vi "Retrieve Question.vi"(8 "error in (no error)":errorcluster, 9 "Difficulty":u32, 10 "Category":string, 11 "Controller in":refnum<class "Controller.lvclass">) -> (0 "error out":errorcluster, 3 "Controller out":refnum<class "Controller.lvclass">)   [LabVIEW 2024, in "Controller.lvlib" / "Controller.lvclass"]
uses:
  Controller.lvclass
  C:/Program Files/National Instruments/LabVIEW 2024/vi.lib/ActorFramework/Actor/Actor.lvclass
  Controller.lvclass/Controller.ctl
  MC Prompt/MC Prompt/MC Prompt.lvclass
  <vilib>/ActorFramework/Actor/Actor.lvclass/Actor.ctl
  <vilib>/ActorFramework/Message Enqueuer/Message Enqueuer.lvclass/Message Enqueuer.ctl
  MC Prompt/MC Prompt/MC Prompt.lvclass/MC Prompt.ctl
  Controller Messages/Question Prompt Display Msg/Question Prompt Display Msg.lvclass/Question Prompt Display Msg.ctl
  MC Screen/Grid Screen Messages/Ensure Cell is Off Msg/Ensure Cell is Off Msg.lvclass/Ensure Cell is Off Msg.ctl
  d7edfcb4-d505-b941-a124-b7699e1ba89e.vi
  <vilib>/ActorFramework/Message Enqueuer/Enqueue.vi
  <vilib>/ActorFramework/Message Enqueuer/Init from Existing Queue.vi
  <vilib>/ActorFramework/Stop Msg/Stop Msg.lvclass
  C:/Program Files/National Instruments/LabVIEW 2024/vi.lib/ActorFramework/Message/Message.lvclass
  Controller Messages/Question Prompt Display Msg/Question Prompt Display Msg.lvclass
  MC Screen/Grid Screen Messages/Ensure Cell is Off Msg/Ensure Cell is Off Msg.lvclass
  <vilib>/ActorFramework/Message Priority Queue/Priority Enqueue.vi
  <vilib>/ActorFramework/Message Enqueuer/Message Enqueuer.lvclass
  <vilib>/ActorFramework/Actor/Actor.lvclass
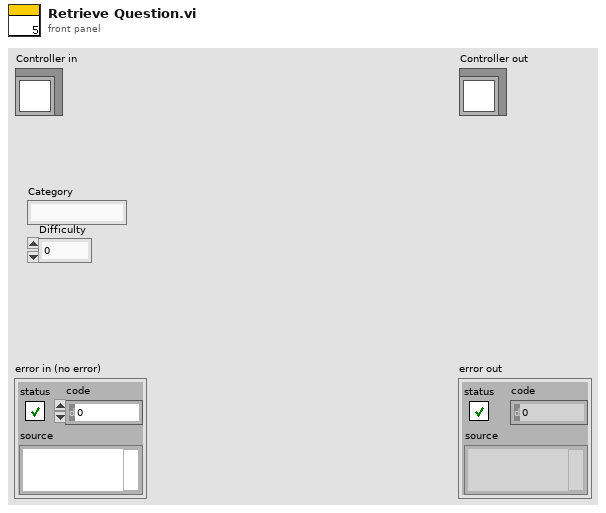
[diagram p1: front panel]
types:
  T1 = map{cluster{"String":string, "String":string}, path}
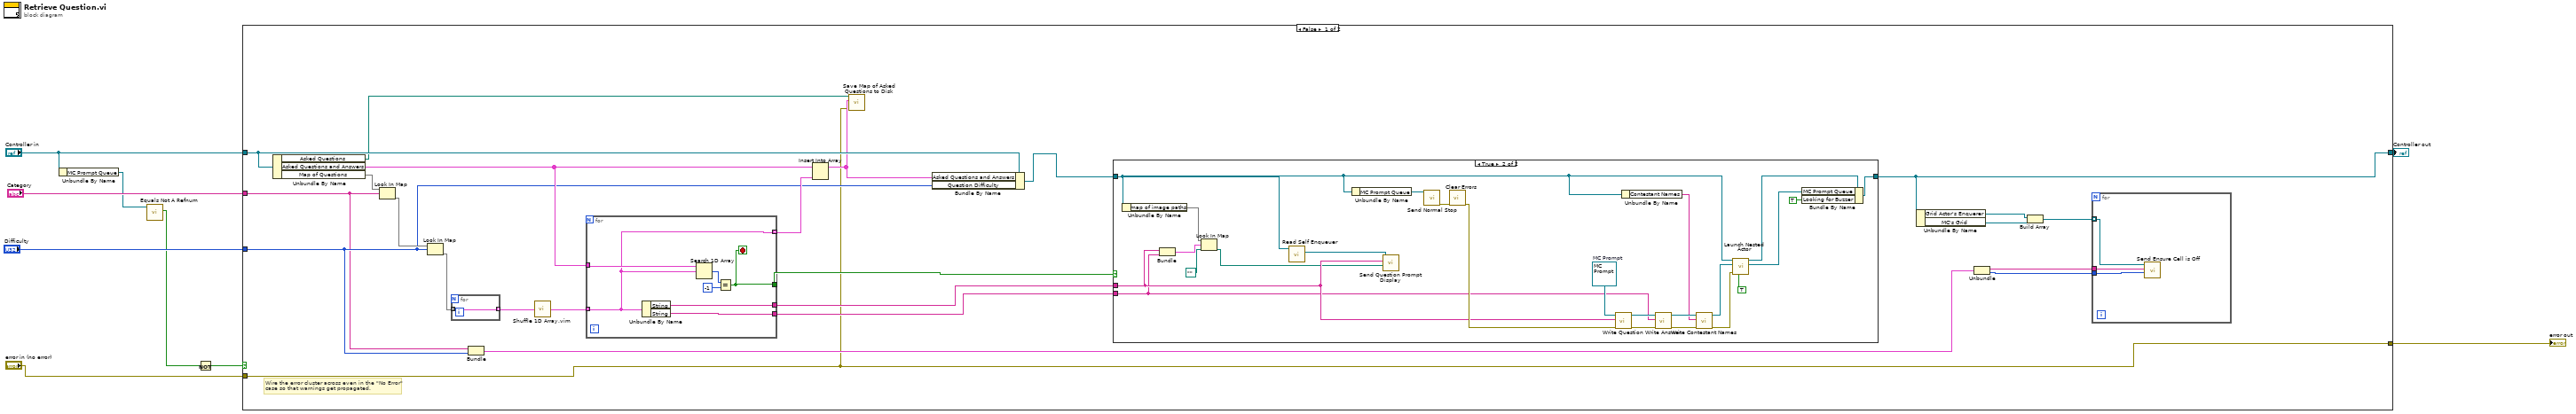
[diagram p0: block diagram]
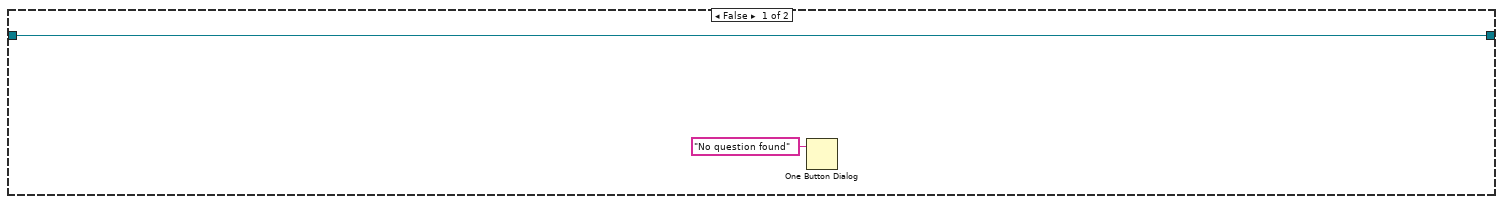
[diagram p2: hidden frame]
diagram:
  n1 = Unbundle By Name("Controller in") -> ("MC Prompt Queue"=w4:refnum<class "Message Enqueuer.lvclass">)
  n2 = call <vilib>:"Equals Not A Refnum.vi"("Message Enqueuer"=w4) -> ("Not a refnum?"=w3:bool)  [unwired: 10 in]
  n3 = Not(x=w3) -> (.not. x?=w1:bool)
  n4 = case shown="False" w1 {
    tunnel: [w10 w71] -> w9
    tunnel: [w20 w72] -> w8
    tunnel: "Controller in" -> [w27 w72]
    tunnel: "Difficulty" -> [w12 _]
    tunnel: "Category" -> [w11 _]
    tunnel: "error in (no error)" -> [w10 w71]
    frame False {
      # "Wire the error cluster across even in the \"No Error\"\ncase so that warnings get propagated."
      n5 = Unbundle By Name(w27) -> ("Asked Questions"=w23:path, "Asked Questions and Answers"=w28:cluster{"String":string, "String":string}[], "Map of Questions"=w33:map{string, map{u32, map{string, string}}})
      n6 = Look In Map(map=w33, key=w11) -> (value=w32:map{u32, map{string, string}})  [unwired: 1 in, 1 out]
      n7 = Look In Map(map=w32, key=w12) -> (value=w31:map{string, string})  [unwired: 1 in, 1 out]
      n8 = for {
        tunnel: w31 -> [w70] mode=indexing
        tunnel: [w70] -> w30 mode=indexing
      }
      n9 = Bundle("Category"=w11, "Difficulty"=w12) -> (w17:cluster{"Category":string, "Difficulty":u32})  [unwired: 1 in]
      n10 = call "Shuffle 1D Array.vim"("array"=w30) -> ("shuffled array"=w29:cluster{"String":string, "String":string}[])  [unwired: 4 in]
      n11 = for {
        tunnel: w29 -> [w63] mode=indexing
        tunnel: w28 -> [w64]
        tunnel: [w67] -> w21
        tunnel: [w66] -> w25
        tunnel: [w65] -> w26
        tunnel: [w63] -> w13 mode=indexing
        stop <- w65 stop-if-true
        n12 = Unbundle By Name(w63) -> ("String"=w67:string, "String"=w66:string)
        n13 = Search 1D Array(1D array=w64, element=w63) -> (index of element=w69:i32)  [unwired: 1 in]
        n14 = Equal?(x=w69, y=-1) -> (x = y?=w65:bool)
      }
      n15 = Insert Into Array(array=w28, new element=w13) -> (w22:cluster{"String":string, "String":string}[])  [unwired: 1 in]
      n16 = call "Save Map of Asked Questions to Disk.vi"("error in (no error)"=w10, "Asked Questions and Answers"=w22, "Asked Questions"=w23) -> ()  [unwired: 9 in]
      n17 = Bundle By Name(cluster=w27, "Asked Questions and Answers"=w22, "Question Difficulty"=w12) -> (w24:refnum<class "Controller.lvclass">)
      n18 = case shown="True" w26 {
        tunnel: w21 -> [_ w43]
        tunnel: w25 -> [_ w42]
        tunnel: w24 -> [w38 w45]
        tunnel: [w38 w54] -> w20
        frame False {
          n19 = One Button Dialog(message="No question found") -> ()  [unwired: 1 in, 1 out]
        }
        frame True {
          w60 = refnum<class "MC Prompt.lvclass"> refnum  # MC Prompt
          n20 = Unbundle By Name(w45) -> ("map of image paths"=w44:T1)
          n21 = Bundle("String"=w43, "String"=w42) -> (w41:cluster{"String":string, "String":string})  [unwired: 1 in]
          n22 = Look In Map(map=w44, key=w41, default value=path "") -> (value=w40:path)  [unwired: 1 out]
          n23 = call <vilib>:"Read Self Enqueuer.vi"("Actor"=w45) -> ("Self Enqueuer"=w53:refnum<class "Message Enqueuer.lvclass">)  [unwired: 10 in]
          n24 = Unbundle By Name(w45) -> ("MC Prompt Queue"=w52:refnum<class "Message Enqueuer.lvclass">)
          n25 = call "Send Question Prompt Display.vi"("Image Path"=w40, "Prompt"=w43, "Message Enqueuer"=w53) -> ()  [unwired: 7 in, 2 out]
          n26 = call <vilib>:"Send Normal Stop.vi"("Message Enqueuer"=w52) -> ("error out"=w51:errorcluster)  [unwired: 10 in]
          n27 = call <vilib>:"Clear Errors.vi"("error in (no error)"=w51) -> ("error out"=w50:errorcluster)  [unwired: 5 in, 1 out]
          n28 = call "Write Question.vi"("error in (no error)"=w50, "Question"=w43, "MC Prompt in"=w60) -> ("error out"=w49:errorcluster, "MC Prompt out"=w61:refnum<class "MC Prompt.lvclass">)  [unwired: 7 in]
          n29 = Unbundle By Name(w45) -> ("Contestant Names"=w57:string[])
          n30 = call "Write Answer.vi"("error in (no error)"=w49, "Answer"=w42, "MC Prompt in"=w61) -> ("error out"=w48:errorcluster, "MC Prompt out"=w59:refnum<class "MC Prompt.lvclass">)  [unwired: 7 in]
          n31 = call "Write Contestant Names.vi"("error in (no error)"=w48, "Contestant Names"=w57, "MC Prompt in"=w59) -> ("error out"=w47:errorcluster, "MC Prompt out"=w58:refnum<class "MC Prompt.lvclass">)  [unwired: 7 in]
          n32 = call <vilib>:"Launch Nested Actor.vi"("Open Actor Core front panel? (F)"=TRUE, "error in (no error)"=w47, "Nested Actor"=w58, "Caller Actor in"=w45) -> ("Nested Actor's Enqueuer"=w55:refnum<class "Message Enqueuer.lvclass">, "Caller Actor out"=w56:refnum<class "Controller.lvclass">)  [unwired: 5 in, 1 out]
          n33 = Bundle By Name(cluster=w56, "MC Prompt Queue"=w55, "Looking for Buzzer"=TRUE) -> (w54:refnum<class "Controller.lvclass">)
        }
      }
      n34 = Unbundle By Name(w20) -> ("Grid Actor's Enquerer"=w19:refnum<class "Message Enqueuer.lvclass">, "MC's Grid"=w18:refnum<class "Message Enqueuer.lvclass">)
      n35 = Unbundle(w17) -> ("Category"=w15:string, "Difficulty"=w14:u32)
      n36 = Build Array(w19, w18) -> (w16:refnum<class "Message Enqueuer.lvclass">[])
      n37 = for {
        tunnel: w16 -> [w35] mode=indexing
        tunnel: w15 -> [w36]
        tunnel: w14 -> [w34]
        n38 = call "Send Ensure Cell is Off.vi"("Difficulty"=w34, "Category"=w36, "Message Enqueuer"=w35) -> ()  [unwired: 7 in, 2 out]
      }
    }
    frame True {
    }
  }
  "error out" <- w9
  "Controller out" <- w8
